vi "Set Key.vi"(6 "key definition":T1, 8 "error in":errorcluster, 9 "key":string, 10 "section":string, 11 "key lookup":variant) -> (0 "error out":errorcluster, 3 "key lookup out":variant)   [LabVIEW 2012, in "configlib.lvlib"]
uses:
  configlib.lvlib
  Key Definition.ctl
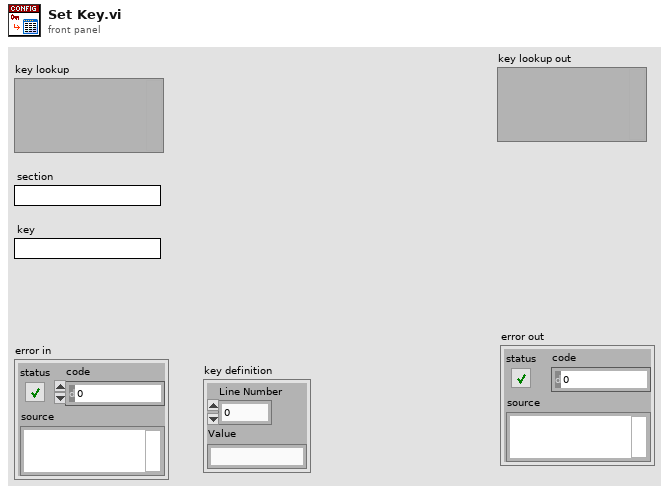
[diagram p1: front panel]
types:
  T1 = typedef "configlib.lvlib/Key Definition.ctl" = cluster{"Line Number":i32, "Value":string}
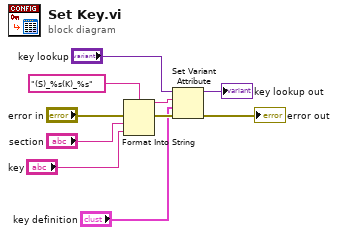
[diagram p0: block diagram]
diagram:
  n1 = Format Into String(format string="(S)_%s(K)_%s", error in="error in", "section", "key") -> (resulting string=w8:string, error out=w7:errorcluster)  [unwired: 1 in]
  n2 = Set Variant Attribute(Variant="key lookup", name=w8, value="key definition", error in=w7) -> (Variant out=→"key lookup out":variant, error out=→"error out":errorcluster)  [unwired: 1 out]
